vi "ProcessDataToServer.vi"(8 "error in (no error)":errorcluster, 9 "data send":T1, 10 "config":T5, 11 "qbus in":refnum<class "Qbus.lvclass">) -> (0 "error out":errorcluster)   [LabVIEW 2017, in "ServerComm.lvlib"]
uses:
  <vilib>/addons/InsightCM/Devices/Shared/Common/ServerComm/ServerComm.lvlib
  <vilib>/addons/InsightCM/Devices/Shared/Common/ServerComm/controls/TcpSendDataConfig.ctl
  <vilib>/addons/InsightCM/Devices/Shared/Common/ServerComm/controls/DataSendParameters.ctl
  <vilib>/addons/InsightCM/Devices/Shared/Common/ServerComm/controls/DataSendBody.ctl
  <vilib>/addons/InsightCM/MessageBus/TcpApi/controls/TcpMessageReference.ctl
  <vilib>/addons/InsightCM/Devices/Shared/Common/ServerComm/controls/DataSendMode.ctl
  <vilib>/addons/InsightCM/MessageBus/Base/controls/IRoutingSource.ctl
  <vilib>/addons/Qbus/Qbus.lvclass
  <vilib>/addons/InsightCM/MessageBus/MessageLibrary/DataStorage/controls/DataStorageCloseEventRequestBody.ctl
  <vilib>/addons/InsightCM/MessageBus/Base/controls/DataSetPacket.ctl
  <vilib>/addons/TraceLogger/TraceLogger.lvlib
  <vilib>/addons/InsightCM/Devices/Shared/Common/DataEvent/DataEvent.lvlib
  <vilib>/addons/InsightCM/Devices/Shared/Common/DataEventCreator/DataEventCreator.lvlib
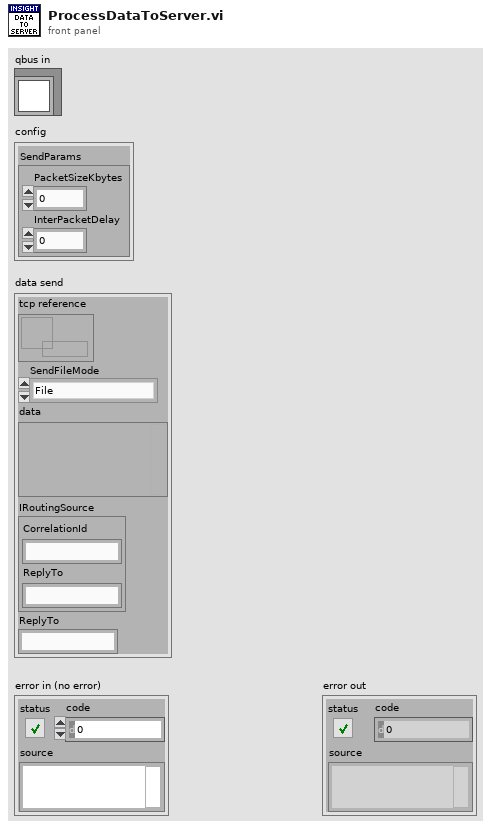
[diagram p1: front panel]
types:
  T1 = typedef "ServerComm.lvlib/DataSendBody.ctl" = cluster{"tcp reference":T2, "SendFileMode":T3, "data":variant, "IRoutingSource":T4, "ReplyTo":string}
  T2 = typedef "TcpMessageReference.ctl" = refnum<data-value>
  T3 = typedef "ServerComm.lvlib/DataSendMode.ctl" = enum16{"File", "InMemoryFile", "Stream", "StreamFileBlock", "ByteArray", "NoOp", "UnknownData"}
  T4 = typedef "IRoutingSource.ctl" = cluster{"CorrelationId":string, "ReplyTo":string}
  T5 = typedef "ServerComm.lvlib/TcpSendDataConfig.ctl" = cluster{"SendParams":T6}
  T6 = typedef "ServerComm.lvlib/DataSendParameters.ctl" = cluster{"PacketSizeKbytes":i32, "InterPacketDelay":i32}
  T7 = typedef "DataStorageCloseEventRequestBody.ctl" = cluster{"EventId":string}
  T8 = typedef "DataSetPacket.ctl" = cluster{"EventId":string, "DataSetId":string, "PacketNumber":i32, "Buffer":u8[], "LastPacket":bool}
  T9 = typedef "DataEvent.lvlib/EventReference.ctl" = refnum<data-value>
  T10 = typedef "DataEvent.lvlib/Event.ctl" = cluster{"DataEvent":T11, "DataSets":T13[], "TrendPoints":T15[], "Alarms":T16[]}
  T11 = typedef "DataEvent.ctl" = cluster{"Id":string, "AssetNodeId":string, "Timestamp":i64, "Props":T12[]}
  T12 = typedef "KeyValuePair.ctl" = cluster{"Key":string, "Value":string}
  T13 = typedef "DataEvent.lvlib/DataSet.ctl" = cluster{"DataSetMetadata":T14, "Values":sgl[], "Values DVR":refnum<data-value>}
  T14 = typedef "DataSetMetadata.ctl" = cluster{"Id":string, "DataEventId":string, "AssetNodeId":string, "Type":string, "T0":i64, "Props":T12[]}
  T15 = typedef "TrendPoint.ctl" = cluster{"TrendPointId":string, "DataEventId":string, "Timestamp":i64, "Value":dbl, "Props":T12[]}
  T16 = typedef "TrendAlarmUpdate.ctl" = cluster{"RuleId":string, "Transition":T17}
  T17 = typedef "TrendAlarmTransition.ctl" = cluster{"At":i64, "Severity":i32, "Value":dbl, "Properties":T12[]}
  T18 = typedef "Message.ctl" = cluster{"Header":T19, "Body":u8[]}
  T19 = typedef "MessageHeader.ctl" = cluster{"MessageName":string, "Timestamp":i64, "CorrelationId":string, "ContentType":string, "RoutingKey":string, "Properties":T12[]}
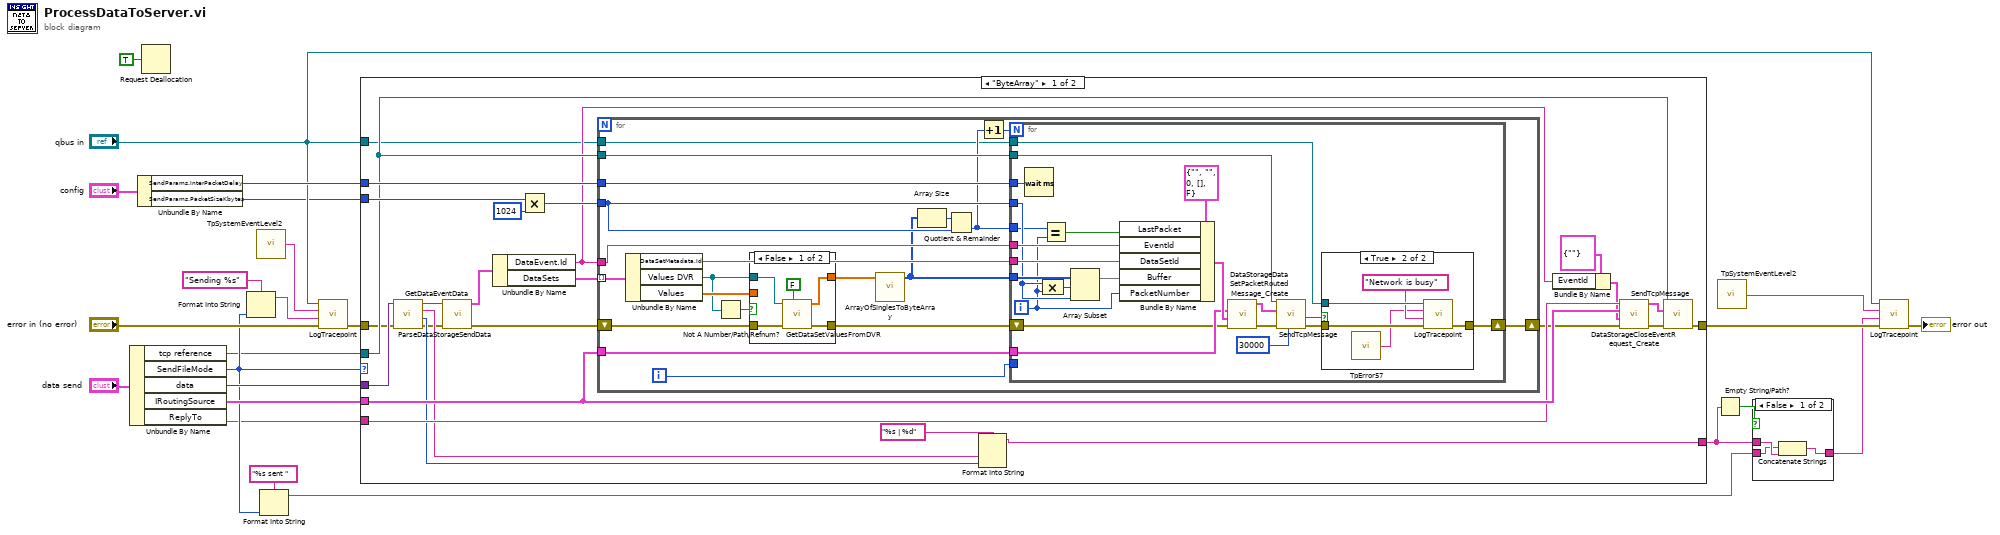
[diagram p0: block diagram]
diagram:
  n1 = Unbundle By Name("data send") -> ("tcp reference"=w7:T2, "SendFileMode"=w12:T3, "data"=w20:variant, "IRoutingSource"=w21:T4, "ReplyTo"=w8:string)
  n2 = Unbundle By Name("config") -> ("SendParams.InterPacketDelay"=w24:i32, "SendParams.PacketSizeKbytes"=w2:i32)
  n3 = Request Deallocation(TRUE ("flag")) -> ()
  n4 = Format Into String(format string="Sending %s", w12) -> (resulting string=w16:string)  [unwired: 2 in, 1 out]
  n5 = call <vilib>:"TpSystemEventLevel2.vi"() -> ("tracepoint name"=w15:string)  [unwired: 5 in]
  n6 = Format Into String(format string="%s sent ", w12) -> (resulting string=w4:string)  [unwired: 2 in, 1 out]
  n7 = call <vilib>:"LogTracepoint.vi"("error in (no error)"="error in (no error)", "log string"=w16, "tracepoint"=w15, "qbus in"="qbus in") -> ("error out"=w17:errorcluster)  [unwired: 6 in, 1 out]
  n8 = case shown="\"ByteArray\"" w12 {
    tunnel: [w42 w106] -> w13
    tunnel: w17 -> [w34 w106]
    tunnel: w7 -> [w41 _]
    tunnel: w21 -> [w39 _]
    tunnel: w24 -> [w50 _]
    tunnel: w2 -> [w48 _]
    tunnel: w20 -> [w35 _]
    tunnel: "qbus in" -> [w29 _]
    tunnel: w8 -> [w38 _]
    tunnel: [w45 _] -> w5
    frame "ByteArray" {
      n9 = call <vilib>:"ParseDataStorageSendData.vi"("error in (no error)"=w34, "body"=w35) -> ("error out"=w27:errorcluster, "block"=w31:i32, "stream id"=w32:string, "event reference"=w28:T9)  [unwired: 4 in, 2 out]
      n10 = call <vilib>:"GetDataEventData.vi"("error in (no error)"=w27, "Data Value Reference in"=w28) -> ("error out"=w25:errorcluster, "Data"=w26:T10)  [unwired: 8 in]
      n11 = Unbundle By Name(w26) -> ("DataEvent.Id"=w33:string, "DataSets"=w44:T13[])
      n12 = Multiply(x=w48, y=1024) -> (x*y=w47:i32)
      n13 = for {
        tunnel: w41 -> [w69]
        tunnel: w29 -> [w58]
        tunnel: w47 -> [w62]
        tunnel: w50 -> [w64]
        tunnel: w39 -> [w68]
        tunnel: w44 -> [w67] mode=indexing
        tunnel: w33 -> [w65]
        shift-right: [w70] -> w30
        shift-left: w25 -> [w52]
        i -> [w59]
        n14 = Unbundle By Name(w67) -> ("DataSetMetadata.Id"=w66:string, "Values DVR"=w53:refnum<data-value>, "Values"=w54:sgl[])
        n15 = Not A Number/Path/Refnum?(number/path/refnum=w53) -> (NaN/Path/Refnum?=w56:bool)
        n16 = case shown="False" w56 {
          tunnel: [w72 w77] -> w55
          tunnel: w54 -> [_ w77]
          tunnel: w53 -> [w75 _]
          tunnel: w52 -> [w74 w76]
          tunnel: [w73 w76] -> w51
          frame False {
            n17 = call <vilib>:"GetDataSetValuesFromDVR.vi"("delete dvr"=FALSE, "error in (no error)"=w74, "values dvr"=w75) -> ("error out"=w73:errorcluster, "values"=w72:sgl[])  [unwired: 7 in]
          }
          frame True {
          }
        }
        n18 = call <vilib>:"ArrayOfSinglesToByteArray.vi"("Values"=w55) -> ("unsigned byte array"=w57:u8[])  [unwired: 4 in]
        n19 = Array Size(array=w57) -> (size(s)=w63:i32)
        n20 = Quotient & Remainder(x=w63, y=w62) -> (floor(x/y)=w60:i32)  [unwired: 1 out]
        n21 = Increment(x=w60) -> (x+1=w61:i32)
        n22 = for {
          N: w61 -> [_]
          tunnel: w58 -> [w80]
          tunnel: w69 -> [w97]
          tunnel: w68 -> [w91]
          tunnel: w66 -> [w90]
          tunnel: w57 -> [w87]
          tunnel: w65 -> [w89]
          shift-right: [w99] -> w70
          shift-left: w51 -> [w88]
          tunnel: w64 -> [w85]
          tunnel: w62 -> [w83]
          tunnel: w60 -> [w82]
          tunnel: w59 -> [_]
          i -> [w78]
          n23 = Wait (ms)(milliseconds to wait=w85) -> ()  [unwired: 1 out]
          n24 = Equal?(x=w82, y=w78) -> (x = y?=w81:bool)
          n25 = Compound Arithmetic op=MULTIPLY(w83, w78) -> (w84:i32)
          n26 = Array Subset(array=w87, index=w84, length=w83) -> (w86:u8[])
          n27 = Bundle By Name(cluster=T8 {"EventId"="", "DataSetId"="", "PacketNumber"=0, "Buffer"=[], "LastPacket"=FALSE} ("DataSet"), "LastPacket"=w81, "EventId"=w89, "DataSetId"=w90, "Buffer"=w86, "PacketNumber"=w78) -> (w94:T8)
          n28 = call <vilib>:"DataStorageDataSetPacketRoutedMessage_Create.vi"("error in (no error)"=w88, "DataSet"=w94, "IRoutingSource"=w91) -> ("error out"=w92:errorcluster, "Message"=w93:T18)  [unwired: 7 in]
          n29 = call <vilib>:"SendTcpMessage.vi"("timeout (5 sec)"=30000, "error in (no error)"=w92, "message"=w93, "connection ID in"=w97) -> ("error out"=w79:errorcluster, "error57"=w98:bool)  [unwired: 5 in, 1 out]
          n30 = case shown="True" w98 {
            tunnel: w79 -> [w100 w105]
            tunnel: [w100 w104] -> w99
            tunnel: w80 -> [_ w103]
            frame False {
            }
            frame True {
              n31 = call <vilib>:"TpError57.vi"() -> ("tracepoint name"=w101:string)  [unwired: 5 in]
              n32 = call <vilib>:"LogTracepoint.vi"("error in (no error)"=w105, "log string"="Network is busy", "tracepoint"=w101, "qbus in"=w103) -> ("error out"=w104:errorcluster)  [unwired: 6 in, 1 out]
            }
          }
        }
      }
      n33 = Format Into String(format string="%s | %d", w32, w31) -> (resulting string=w45:string)  [unwired: 2 in, 1 out]
      n34 = Bundle By Name(cluster=T7 {"EventId"=""} ("Body"), "EventId"=w33) -> (w36:T7)
      n35 = call <vilib>:"DataStorageCloseEventRequest_Create.vi"("error in (no error)"=w30, "DataStorageCloseEventRequest"=w36, "IRoutingSource"=w39, "ReplyTo"=w38) -> ("error out"=w43:errorcluster, "Message"=w40:T18)  [unwired: 6 in]
      n36 = call <vilib>:"SendTcpMessage.vi"("error in (no error)"=w43, "message"=w40, "connection ID in"=w41) -> ("error out"=w42:errorcluster)  [unwired: 6 in, 2 out]
    }
    frame Default {
    }
  }
  n37 = Empty String/Path?(string/path=w5) -> (empty?=w6:bool)
  n38 = call <vilib>:"TpSystemEventLevel2.vi"() -> ("tracepoint name"=w10:string)  [unwired: 5 in]
  n39 = case shown="False" w6 {
    tunnel: w5 -> [w109 _]
    tunnel: w4 -> [w108 w110]
    tunnel: [w107 w110] -> w3
    frame False {
      n40 = Concatenate Strings(w108, w109) -> (w107:string)
    }
    frame True {
    }
  }
  n41 = call <vilib>:"LogTracepoint.vi"("error in (no error)"=w13, "log string"=w3, "tracepoint"=w10, "qbus in"="qbus in") -> ("error out"=→"error out":errorcluster)  [unwired: 6 in, 1 out]
